vi "Drivetrain Set.vi"(1 "Drivetrain Control":T1={"axis 1 (x)"=0.0, "axis 2 (y)"=0.0, "Mode"=enum."Manual", "heading target"=0.0, "steer axis"=0.0, "omni?"=FALSE, "Low Gear?"=FALSE, "distance target"={"x"=0.0, "y"=0.0}, "PID Params"={"X Dist"={"PID gains"={"proportional gain (Kc)"=1.0, "integral time (Ti, min)"=0.0, "derivative time (Td, min)"=0.0}, "output range"={"output high"=1.0, "output low"=-1.0}}, "Y Dist"={"PID gains"={"proportional gain (Kc)"=1.0, "integral time (Ti, min)"=0.0, "derivative time (Td, min)"=0.0}, "output range"={"output high"=1.0, "output low"=-1.0}}}, "Coast"=FALSE} {"PID Params"."Y Dist"."output range"."output low" format="%.2f"; "PID Params"."Y Dist"."output range"."output high" format="%.2f"; "PID Params"."Y Dist"."PID gains"."derivative time (Td, min)" format="%.3f"; "PID Params"."Y Dist"."PID gains"."integral time (Ti, min)" format="%.3f"; "PID Params"."Y Dist"."PID gains"."proportional gain (Kc)" format="%.3f"; "PID Params"."X Dist"."output range"."output low" format="%.2f"; "PID Params"."X Dist"."output range"."output high" format="%.2f"; "PID Params"."X Dist"."PID gains"."derivative time (Td, min)" format="%.3f"; "PID Params"."X Dist"."PID gains"."integral time (Ti, min)" format="%.3f"; "PID Params"."X Dist"."PID gains"."proportional gain (Kc)" format="%.3f"}) -> ()   [LabVIEW 2013]
uses:
  Drivetrain Control.ctl
  DT Mode.ctl
  Distance Drive Result.ctl
  Common Code/Change Detect Int.vi
  Robot Global Data.vi
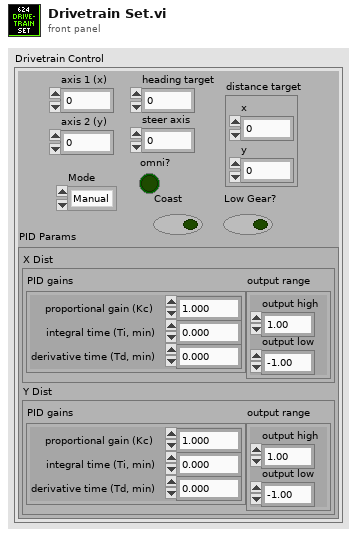
[diagram p1: front panel]
types:
  T1 = typedef "Drivetrain Control.ctl" = cluster{"axis 1 (x)":dbl, "axis 2 (y)":dbl, "Mode":T2, "heading target":dbl, "steer axis":dbl, "omni?":bool, "Low Gear?":bool, "distance target":cluster{"x":dbl, "y":dbl}, "PID Params":cluster{"X Dist":cluster{"PID gains":cluster{"proportional gain (Kc)":dbl, "integral time (Ti, min)":dbl, "derivative time (Td, min)":dbl}, "output range":cluster{"output high":dbl, "output low":dbl}}, "Y Dist":cluster{"PID gains":cluster{"proportional gain (Kc)":dbl, "integral time (Ti, min)":dbl, "derivative time (Td, min)":dbl}, "output range":cluster{"output high":dbl, "output low":dbl}}}, "Coast":bool}
  T2 = typedef "DT Mode.ctl" = enum16{"Manual", "Gyro Steer", "Distance Drive", "Fieldcentric", "Roll Maneuver", "Alt Roll Maneuver"}
  T3 = typedef "Distance Drive Result.ctl" = cluster{"Finished":bool, "distance target":cluster{"x":dbl, "y":dbl}, "Heading Target":dbl, "X Check":bool, "Y Check":bool, "X Dist":dbl, "Y Dist":dbl}
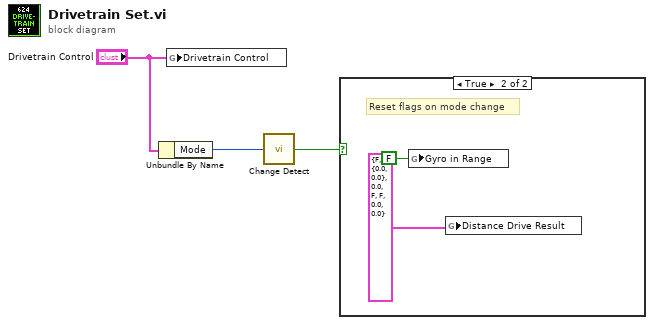
[diagram p0: block diagram]
diagram:
  n1 = Unbundle By Name("Drivetrain Control") -> ("Mode"=w3:T2)
  n2 = global write "Robot Global Data.vi" "Drivetrain Control"("Drivetrain Control") -> ()
  n3 = call-poly "Change Detect.vi"("In"=w3) -> ("Changed?"=w2:bool)
  n4 = case shown="True" w2 {
    frame False {
    }
    frame True {
      # "Reset flags on mode change"
      n5 = global write "Robot Global Data.vi" "Gyro in Range"(FALSE ("Distance Drive Finished?")) -> ()
      n6 = global write "Robot Global Data.vi" "Distance Drive Result"(T3 {"Finished"=FALSE, "distance target"={"x"=0.0, "y"=0.0}, "Heading Target"=0.0, "X Check"=FALSE, "Y Check"=FALSE, "X Dist"=0.0, "Y Dist"=0.0} ("Distance Drive Result")) -> ()
    }
  }
